vi "FPGA Interface - 9035.vi"(6 "FIFO Cluster":T1, 8 "FPGA VI Reference":refnum<k20>, 9 "Name Cluster":T2, 10 "RT Main Message Handler":refnum<queue>, 11 "Logging?":refnum<vi>) -> ()   [LabVIEW 2017]
uses:
  Support Vis/Message Queue/Message Cluster.ctl
  Controls/Logging names.ctl
  <vilib>/Platform/TimedLoop/XDataNode/timing_clust.ctl
  <vilib>/Platform/TimedLoop/XDataNode/nitl_modes.ctl
  <vilib>/Platform/TimedLoop/XDataNode/wakeup.ctl
  Controls/Manual Control.ctl
  Globals/RT/Global - Valves.vi
  <vilib>/Utility/error.llb/Error Cluster From Error Code.vi
  <vilib>/rvi/errors/niLvFpgaAdjustHostInterfaceError.vi
  <vilib>/platform/TimedLoop/XDataNode/XDataNode.xnode
  <vilib>/rvi/interface/nirviReadWriteControl/nirviReadWriteControl.xnode
  <vilib>/rvi/interface/nirviMethod/nirviMethod.xnode
  <vilib>/FPGAPlugInAG/Dynamic/niLvFpga_ReadFifo_Dynamic.vi
  <vilib>/rvi/errors/niLvFpgaMergeErrorWithErrorCode.vi
  <vilib>/Platform/TimedLoop/XDataNode/XDNodeRunTimeDep.lvlib
  Support Vis/Message Queue/Message Queue.lvlib
  NiFpgaLv.dll
  <vilib>/rvi/interface/Simulation/niFpgaSimulationCallBeginRW.vi
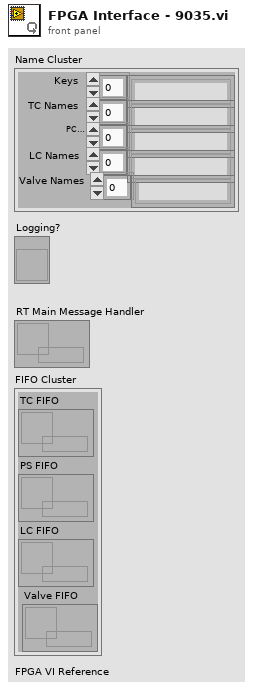
[diagram p1: front panel]
types:
  T1 = cluster{"TC FIFO":refnum<k33>, "PS FIFO":refnum<k33>, "LC FIFO":refnum<k33>, "Valve FIFO":refnum<k33>}
  T2 = typedef "Logging names.ctl" = cluster{"Keys":string[], "TC Names":string[], "PC Names":string[], "LC Names":string[], "Valve Names":string[]}
  T3 = enum16{"Manual", "Standby", "Automated Sequence", "Automated Sequence End", "Emergency"}
  T4 = cluster{"Elements Remaining":u32, "Elements Remaining":u32, "Elements Remaining":u32}
  T5 = typedef "XDNodeRunTimeDep.lvlib/timing_clust.ctl" = cluster{"Expected End [f-1]":u64, "Actual End [f-1]":u64, "Finished Late? [f-1]":bool, "Expected End [i-1]":u64, "Actual End [i-1]":u64, "Finished Late? [i-1]":bool, "Expected Start [i]":u64, "Actual Start [i]":u64, "Expected Start [f]":u64, "Actual Start [f]":u64, "Source Name":string, "Structure Name":string, "Period":i64, "Deadline":i64, "Offset":i64, "Start":i64, "Priority":i32, "Timeout":i32, "Mode":T6, "Wakeup Reason":T7, "Error":errorcluster, "Source Type":string, "Secondary Source Type":string, "Global End Time":u64, "Global Start Time":u64, "Frame Duration":u64, "Iteration Duration":u64, "Assigned CPU":i32, "I/O Scan Engine Mode":u32}
  T6 = typedef "XDNodeRunTimeDep.lvlib/nitl_modes.ctl" = enum32{"No Change", "Process missed periods, maintain original phase", "Discard missed periods, maintain original phase", "Process missed periods, ignore original phase", "Discard missed periods, ignore original phase"}
  T7 = typedef "XDNodeRunTimeDep.lvlib/wakeup.ctl" = enum32{"Normal", "Aborted", "Asynchronous wakeup", "Timing source error", "Timed loop error", "Timeout"}
  T8 = cluster{"Unpowered State":u8, "Output Port":u8, "Emergency State":u8, "Blank Button":bool, "Open Time [ms]":fxp<+/-,18,18>, "Close Time [ms]":fxp<+/-,18,18>, "Active":bool}[]
  T9 = typedef "Manual Control.ctl" = cluster{"Actuator Settings":cluster{"Actuator Name":string, "Unpowered State":i16, "Output Port":u32, "Emergency State":i16, "Blank Button":bool, "Open Time [ms]":i16, "Close Time [ms]":i16}[]}
  T10 = cluster{"Actuator Name":string, "Unpowered State":i16, "Output Port":u32, "Emergency State":i16, "Blank Button":bool, "Open Time [ms]":i16, "Close Time [ms]":i16}[]
  T11 = cluster{"Actuator Name":string, "Unpowered State":i16, "Output Port":u32, "Emergency State":i16, "Blank Button":bool, "Open Time [ms]":i16, "Close Time [ms]":i16}
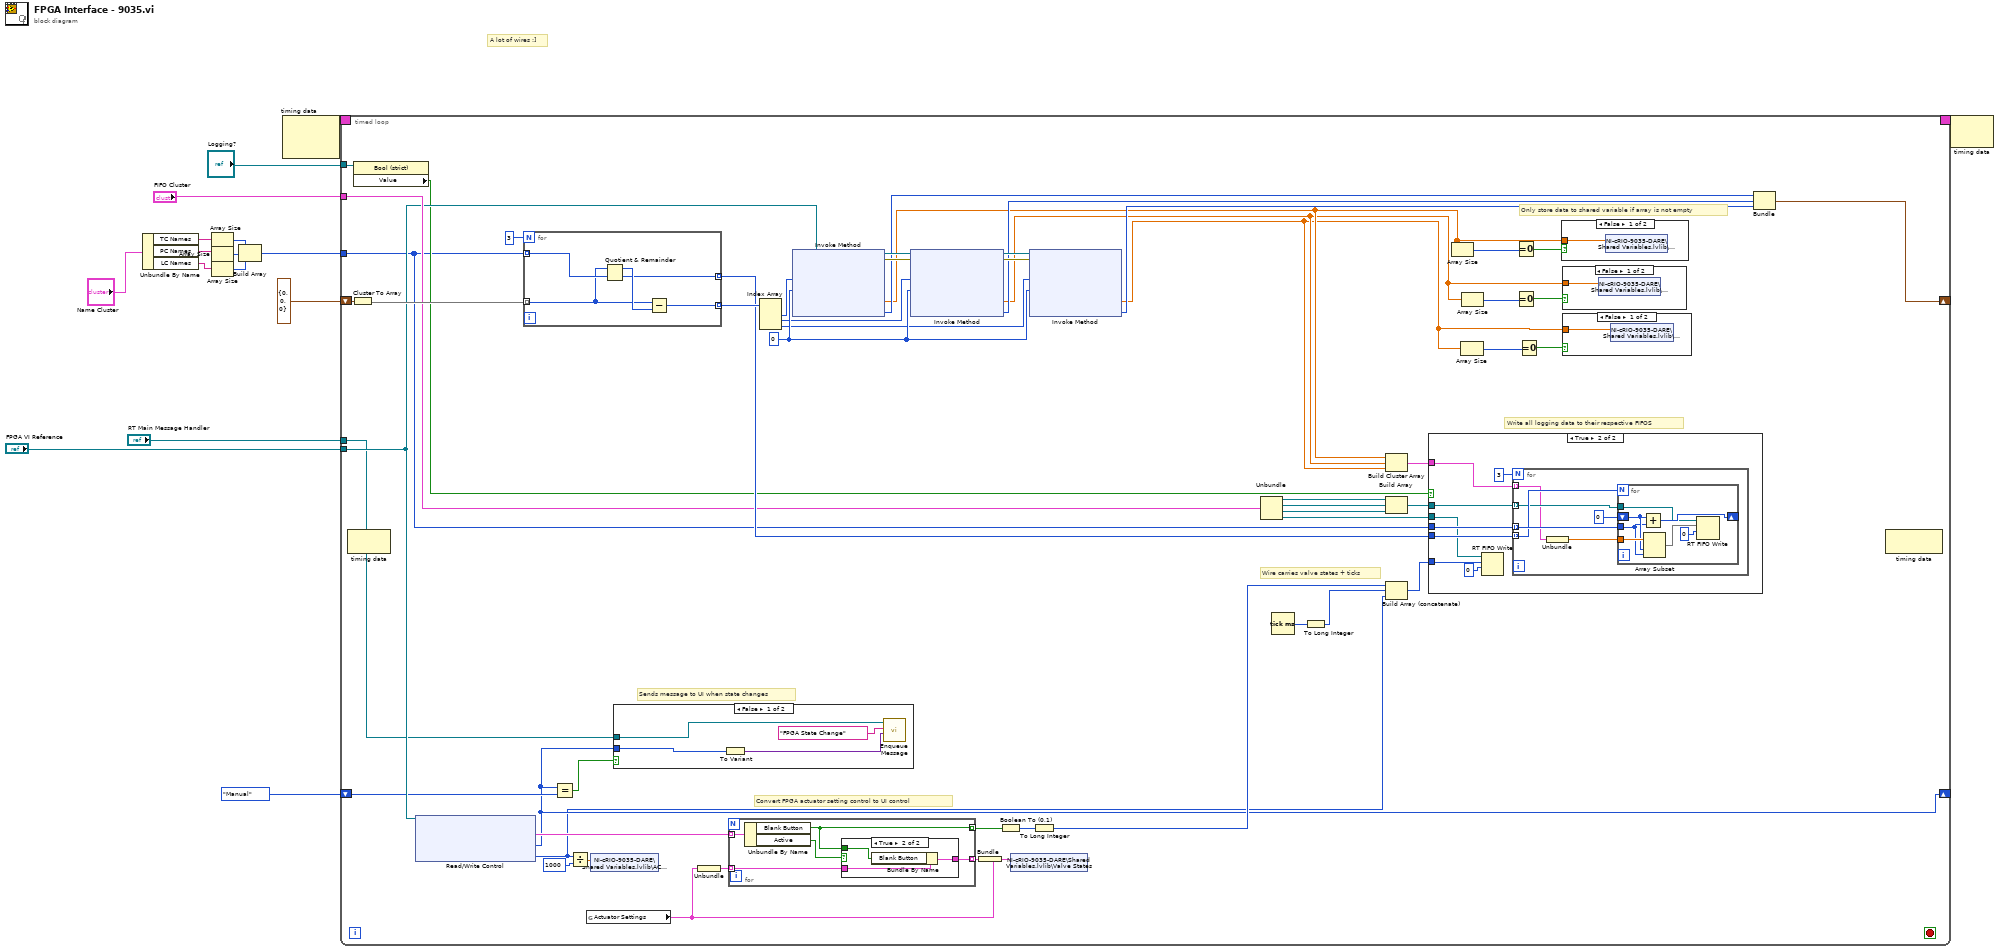
[diagram p0: block diagram]
diagram:
  # "A lot of wires :]"
  n1 = Unbundle By Name("Name Cluster") -> ("TC Names"=w8:string[], "PC Names"=w7:string[], "LC Names"=w6:string[])
  n2 = Array Size(array=w8) -> (size(s)=w3:i32)
  n3 = Array Size(array=w7) -> (size(s)=w5:i32)
  n4 = Array Size(array=w6) -> (size(s)=w4:i32)
  n5 = Build Array(w3, w5, w4) -> (w2:i32[])
  n6 = node-c288() -> (w16:T5)  [unwired: 2 in]
  n7 = timed-loop {
    tunnel: "FPGA VI Reference" -> [w41]
    shift-right: [w63] -> _
    shift-left: T4 {"Elements Remaining"=0, "Elements Remaining"=0, "Elements Remaining"=0} -> [w61]
    tunnel: "FIFO Cluster" -> [w53]
    timing: w16 -> [_]
    timing-out: [_] -> w15
    shift-right: [w20] -> _
    shift-left: T3."Manual" ("FPGA States") -> [w34]
    tunnel: "RT Main Message Handler" -> [w32]
    tunnel: "Logging?" -> [w25]
    tunnel: w2 -> [w21]
    stop <- _ stop-if-true
    w67 = 0 ("Timeout (ms)")
    # "Convert FPGA actuator setting control to UI control"
    # "Wire carries valve states + ticks"
    # "Write all logging data to their respective FIFOS"
    # "Only store data to shared variable if array is not empty"
    # "Sends message to UI when state changes"
    n8 = node-c288() -> ()  [unwired: 1 in, 1 out]
    n9 = Cluster To Array(cluster=w61) -> (array=w60:u32[])
    n10 = property class="Bool (strict)"(reference=w25) -> ("Value"=w26:bool)  [unwired: 1 in, 2 out]
    n11 = xnode "Read/Write Control"("FPGA VI Reference In"=w41) -> ("Actuator Settings"=w24:T8, "FPGA States"=w20:T3, "Automated Sequence Timer"=w19:i32)  [unwired: 1 in, 2 out]
    n12 = for {
      N: 3 -> [_]
      tunnel: w60 -> [w113] mode=indexing
      tunnel: w21 -> [w115] mode=indexing
      tunnel: [w112] -> w59 mode=indexing
      tunnel: [w111] -> w54 mode=indexing
      n13 = Quotient & Remainder(x=w113, y=w115) -> (x-y*floor(x/y)=w114:u32, floor(x/y)=w111:u32)
      n14 = Subtract(x=w113, y=w114) -> (x-y=w112:u32)
    }
    n15 = Equal?(x=w20, y=w34) -> (x = y?=w33:bool)
    n16 = Divide(x=w19, y=1000) -> (x/y=w39:dbl)
    n17 = global read "Global - Valves.vi" "Actuator Settings"() -> (w27:T9)
    n18 = shared-variable "NI-cRIO-9035-DARE\\Shared Variables.lvlib\\AC Timer"(w39) -> ()  [unwired: 1 in, 1 out]
    n19 = case shown="False" w33 {
      tunnel: w32 -> [w83 _]
      tunnel: w20 -> [w82 _]
      frame False {
        n20 = To Variant(anything=w82) -> (Variant=w81:variant)
        n21 = call "Enqueue Message.vi"("Message Data"=w81, "Message"="FPGA State Change", "Message Queue"=w83) -> ()  [unwired: 7 in, 2 out]
      }
      frame True {
      }
    }
    n22 = Unbundle(w27) -> ("Actuator Settings"=w30:T10)
    n23 = for {
      tunnel: w24 -> [w76] mode=indexing
      tunnel: [w72] -> w31 mode=indexing
      tunnel: w30 -> [w75] mode=indexing
      tunnel: [w73] -> w29 mode=indexing
      n24 = Unbundle By Name(w76) -> ("Blank Button"=w72:bool, "Active"=w74:bool)
      n25 = case shown="True" w74 {
        tunnel: w75 -> [w77 w80]
        tunnel: w72 -> [_ w79]
        tunnel: [w77 w78] -> w73
        frame False {
        }
        frame True {
          n26 = Bundle By Name(cluster=w80, "Blank Button"=w79) -> (w78:T11)
        }
      }
    }
    n27 = Index Array(array=w59) -> (element #1=w58:u32, element #2=w57:u32, element #3=w56:u32)  [unwired: 3 in]
    n28 = xnode "Invoke Method"("FPGA VI Reference In"=w41, "Number of Elements"=w58, "Timeout (ms)"=w67) -> ("FPGA VI Reference Out"=w71:refnum<k20>, "error out"=w70:errorcluster, "Data"=w46:sgl[], "Elements Remaining"=w66:u32)  [unwired: 1 in]
    n29 = xnode "Invoke Method"("FPGA VI Reference In"=w71, "error in"=w70, "Number of Elements"=w57, "Timeout (ms)"=w67) -> ("FPGA VI Reference Out"=w69:refnum<k20>, "error out"=w68:errorcluster, "Data"=w23:sgl[], "Elements Remaining"=w65:u32)
    n30 = Bundle(cluster=w27, "Actuator Settings"=w29) -> (w28:T9)
    n31 = Boolean To (0,1)(Boolean=w31) -> (0, 1=w37:i16[])
    n32 = shared-variable "NI-cRIO-9035-DARE\\Shared Variables.lvlib\\Valve States"(w28) -> ()  [unwired: 1 in, 1 out]
    n33 = xnode "Invoke Method"("FPGA VI Reference In"=w69, "error in"=w68, "Number of Elements"=w56, "Timeout (ms)"=w67) -> ("Data"=w22:sgl[], "Elements Remaining"=w64:u32)  [unwired: 2 out]
    n34 = To Long Integer(number=w37) -> (32bit integer=w36:i32[])
    n35 = Unbundle(w53) -> ("TC FIFO"=w52:refnum<k33>, "PS FIFO"=w51:refnum<k33>, "LC FIFO"=w50:refnum<k33>, "Valve FIFO"=w38:refnum<k33>)
    n36 = Tick Count (ms)() -> (millisecond timer value=w18:u32)
    n37 = To Long Integer(number=w18) -> (32bit integer=w17:i32)
    n38 = Build Cluster Array(w46, w23, w22) -> (w55:cluster{"Data":sgl[]}[])
    n39 = Build Array(w52, w51, w50) -> (w49:refnum<k33>[])
    n40 = Build Array (concatenate)(w36, w17, w19) -> (w35:i32[])
    n41 = case shown="True" w26 {
      tunnel: w55 -> [_ w86]
      tunnel: w21 -> [_ w92]
      tunnel: w54 -> [_ w91]
      tunnel: w49 -> [_ w90]
      tunnel: w38 -> [_ w88]
      tunnel: w35 -> [_ w89]
      frame False {
      }
      frame True {
        n42 = RT FIFO Write(0:w88, 1:w89, 2:0 ("timeout in ms (0)")) -> ()  [unwired: 2 in, 4 out]
        n43 = for {
          N: 3 -> [_]
          tunnel: w86 -> [w94] mode=indexing
          tunnel: w92 -> [w98] mode=indexing
          tunnel: w91 -> [w96] mode=indexing
          tunnel: w90 -> [w95] mode=indexing
          n44 = Unbundle(w94) -> ("Data"=w93:sgl[])
          n45 = for {
            N: w96 -> [_]
            tunnel: w93 -> [w105]
            tunnel: w98 -> [w101]
            shift-right: [w100] -> _
            shift-left: 0 ("index") -> [w102]
            tunnel: w95 -> [w99]
            n46 = Add(x=w102, y=w101) -> (x+y=w100:i32)
            n47 = Array Subset(array=w105, index=w102, length=w101) -> (w104:sgl[])
            n48 = RT FIFO Write(0:w99, 1:w104, 2:0 ("timeout in ms (0)")) -> ()  [unwired: 2 in, 4 out]
          }
        }
      }
    }
    n49 = Array Size(array=w46) -> (size(s)=w48:i32)
    n50 = Array Size(array=w22) -> (size(s)=w43:i32)
    n51 = Array Size(array=w23) -> (size(s)=w44:i32)
    n52 = Equal To 0?(x=w48) -> (x = 0?=w47:bool)
    n53 = Equal To 0?(x=w44) -> (x = 0?=w45:bool)
    n54 = Equal To 0?(x=w43) -> (x = 0?=w42:bool)
    n55 = case shown="False" w47 {
      tunnel: w46 -> [w110 _]
      frame False {
        n56 = shared-variable "NI-cRIO-9035-DARE\\Shared Variables.lvlib\\TC Data"(w110) -> ()  [unwired: 1 in, 1 out]
      }
      frame True {
      }
    }
    n57 = case shown="False" w45 {
      tunnel: w23 -> [w109 _]
      frame False {
        n58 = shared-variable "NI-cRIO-9035-DARE\\Shared Variables.lvlib\\PS Data"(w109) -> ()  [unwired: 1 in, 1 out]
      }
      frame True {
      }
    }
    n59 = case shown="False" w42 {
      tunnel: w22 -> [w108 _]
      frame False {
        n60 = shared-variable "NI-cRIO-9035-DARE\\Shared Variables.lvlib\\LC Data"(w108) -> ()  [unwired: 1 in, 1 out]
      }
      frame True {
      }
    }
    n61 = Bundle("Elements Remaining"=w66, "Elements Remaining"=w65, "Elements Remaining"=w64) -> (w63:T4)  [unwired: 1 in]
    n62 = node-c288() -> ()  [unwired: 1 in, 1 out]
  }
  n63 = node-c288(w15) -> ()  [unwired: 1 out]
